vi "python.vi"() -> ()   [LabVIEW 2011]
panel:
  out "String":string
  out "Raw Python String Output":string
  out "error out":errorcluster
  out "Standard Error":string
  out "Return Code":i32
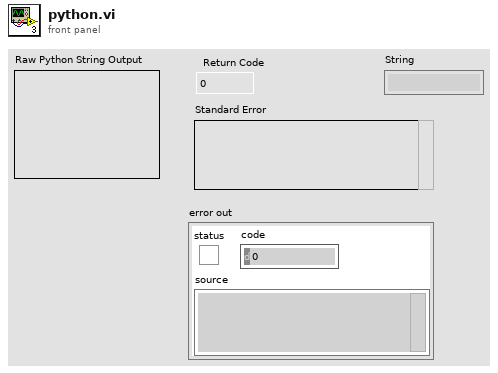
[diagram p1: front panel]
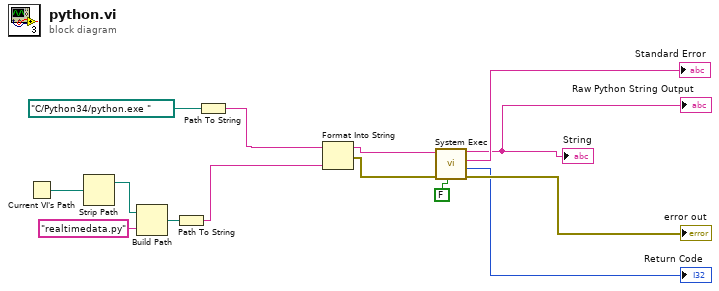
[diagram p0: block diagram]
diagram:
  n1 = Current VI's Path() -> (path=w10:path)
  n2 = Strip Path(path=w10) -> (stripped path=w9:path)  [unwired: 1 out]
  n3 = Build Path(base path=w9, name or relative path="realtimedata.py" ("Path to Function")) -> (appended path=w11:path)
  n4 = Path To String(path=w11) -> (string=w8:string)
  n5 = Path To String(path=path "C:/Python34/python.exe ") -> (string=w13:string)
  n6 = Format Into String(initial string=w13, w8) -> (resulting string=w2:string, error out=w3:errorcluster)  [unwired: 2 in]
  n7 = call <vilib>:"System Exec.vi"("run minimized? (F)"=FALSE, "error in (no error)"=w3, "command line"=w2) -> ("error out"=→"error out":errorcluster, "return code"=→"Return Code":i32, "standard error"=→"Standard Error":string, "standard output"=→"Raw Python String Output" →"String":string)  [unwired: 5 in]
